vi "SetExtTrigSD.vi"   [LabVIEW 2015]
uses:
  DLL/ESLSCDLL.dll
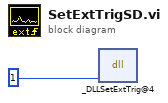
[diagram p0: block diagram]
diagram:
  n1 = dll-call lib="G:/SD/TRANCON/DLL/ESLSCDLL.dll" fn="_DLLSetExtTrig@4" ("lwlscdll.dll:DLLSetExtTrig")("drv"=u32 1) -> ()  [unwired: 5 in, 2 out]
